vi "Write Bounds.vi"(8 "error in (no error)":errorcluster, 10 "Rect":T1, 11 "Rectangle Mask in":refnum<class "Rectangle Mask.lvclass">) -> (0 "error out":errorcluster, 3 "Rectangle Mask out":refnum<class "Rectangle Mask.lvclass">)   [LabVIEW 2016, in "Rectangle Mask.lvclass"]
uses:
  Rectangle Mask.lvclass
  <vilib>/Utility/miscctls.llb/LVRectTypeDef.ctl
  Rectangle Mask.lvclass/Rectangle Mask.ctl
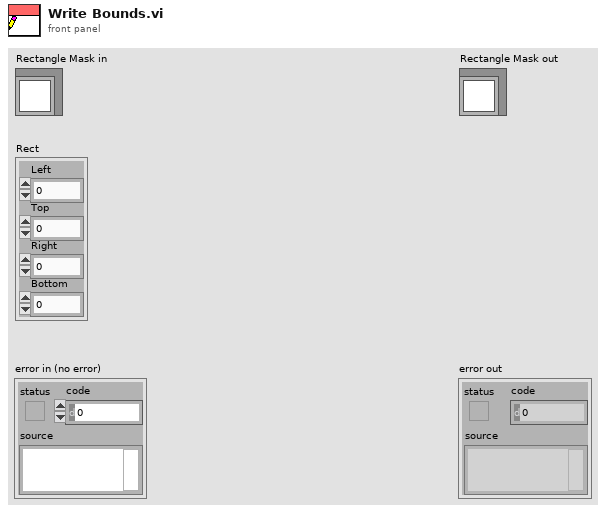
[diagram p1: front panel]
types:
  T1 = typedef "LVRectTypeDef.ctl" = cluster{"Left":i16, "Top":i16, "Right":i16, "Bottom":i16}
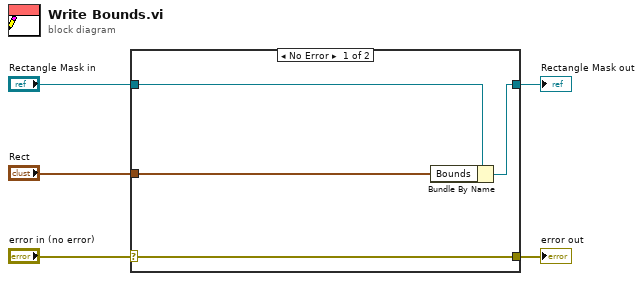
[diagram p0: block diagram]
diagram:
  n1 = case shown="No Error" "error in (no error)" {
    selector: "error in (no error)" -> [w9 w10]
    tunnel: [w9 w10] -> w4
    tunnel: [w7 w11] -> w2
    tunnel: "Rectangle Mask in" -> [w8 w11]
    tunnel: "Rect" -> [w6 _]
    frame No Error {
      n2 = Bundle By Name(cluster=w8, "Bounds"=w6) -> (w7:refnum<class "Rectangle Mask.lvclass">)
    }
    frame Error {
    }
  }
  "error out" <- w4
  "Rectangle Mask out" <- w2
